vi "Get Arm.vi"(8 "error in (no error)":errorcluster, 11 "KUKA youBot host in":refnum<class "NI_Robotics_KUKA youBot Host Interface.lvclass">) -> (0 "error out":errorcluster, 2 "KUKA youBot arm out":refnum<class "NI_Robotics_KUKA youBot Arm.lvclass">, 3 "KUKA youBot host out":refnum<class "NI_Robotics_KUKA youBot Host Interface.lvclass">)   [LabVIEW 2017, in "NI_Robotics_KUKA youBot Host.lvlib" / "NI_Robotics_KUKA youBot Host Interface.lvclass"]
doc: "Gets an arm instance from the KUKA youBot indicated by the arm index."
uses:
  <vilib>/robotics/KUKA youBot/Host Interface/NI_Robotics_KUKA youBot Host Interface.lvclass
  <vilib>/robotics/KUKA youBot/Basic Device/Arm/NI_Robotics_KUKA youBot Arm.lvclass
  <vilib>/robotics/KUKA youBot/Host Interface/NI_Robotics_KUKA youBot Host Interface.lvclass/NI_Robotics_KUKA youBot Host Interface.ctl
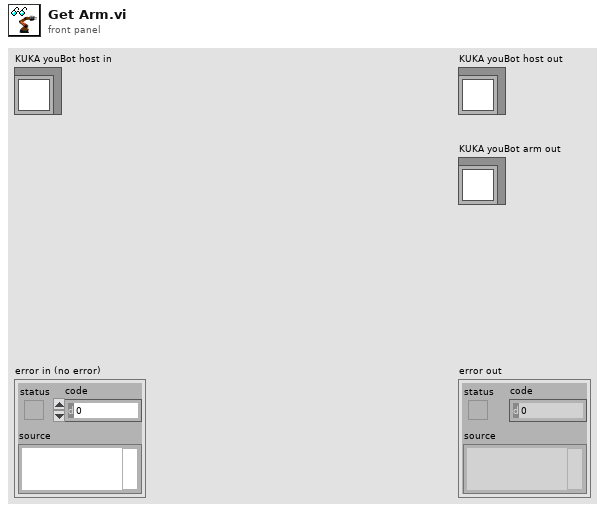
[diagram p1: front panel]
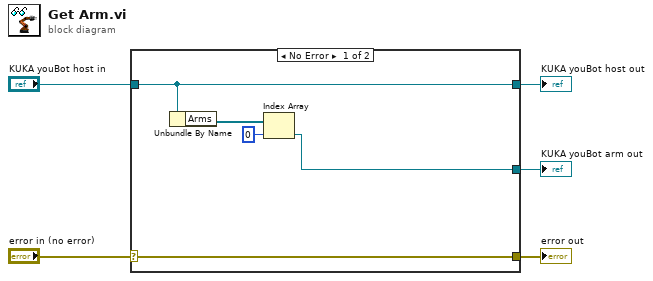
[diagram p0: block diagram]
diagram:
  n1 = case shown="No Error" "error in (no error)" {
    selector: "error in (no error)" -> [w10 w11]
    tunnel: [w10 w11] -> w4
    tunnel: [w9 w12] -> w2
    tunnel: "KUKA youBot host in" -> [w9 w12]
    tunnel: [w7 _] -> w1
    frame No Error {
      n2 = Unbundle By Name(w9) -> ("Arms"=w8:refnum<class "NI_Robotics_KUKA youBot Arm.lvclass">[])
      n3 = Index Array(array=w8, index=0) -> (element=w7:refnum<class "NI_Robotics_KUKA youBot Arm.lvclass">)
    }
    frame Error {
    }
  }
  "error out" <- w4
  "KUKA youBot host out" <- w2
  "KUKA youBot arm out" <- w1
